vi "Read State com.vi"(8 "error in (no error)":errorcluster, 11 "Master CR in":refnum<class "Master CR.lvclass">) -> (0 "error out":errorcluster, 2 "State com":T1, 3 "Master CR out":refnum<class "Master CR.lvclass">)   [LabVIEW 2021, in "Master CR.lvclass"]
uses:
  Master CR.lvclass
  ctl/Master CR state.ctl
  ctl/CR_Core_State.ctl
  Master CR.lvclass/Master CR.ctl
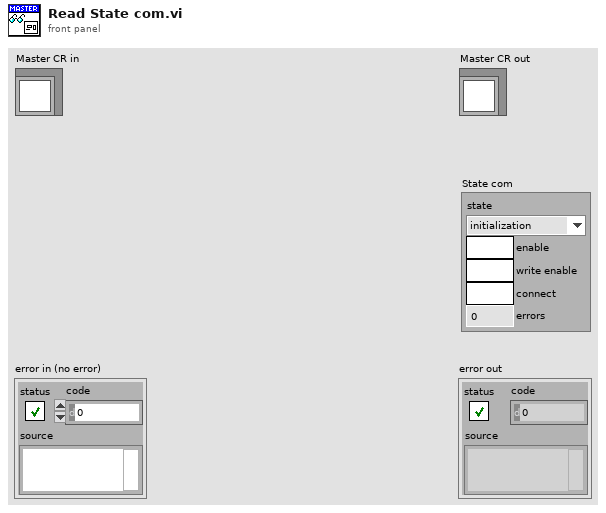
[diagram p1: front panel]
types:
  T1 = typedef "Master CR.lvclass/Master CR state.ctl" = cluster{"state":T2, "enable":bool, "write enable":bool, "connect":bool, "errors":i32}
  T2 = typedef "Master CR.lvclass/CR_Core_State.ctl" = enum8{"initialization", "redefine", "standby", "ping", "connect", "wait to reconnect", "wait to reset timeout", "configure", "requests", "close connection", "stop"}
  T3 = typedef "Master CR.lvclass/MB state.ctl" = cluster{"state":T4, "enable":bool, "write enable":bool, "connect":bool, "errors":i32}
  T4 = typedef "Master CR.lvclass/MB_TCP_State.ctl" = enum8{"initialization", "redefine", "standby", "ping", "connect", "wait to reconnect", "wait to reset timeout", "configure", "requests", "close connection", "stop"}
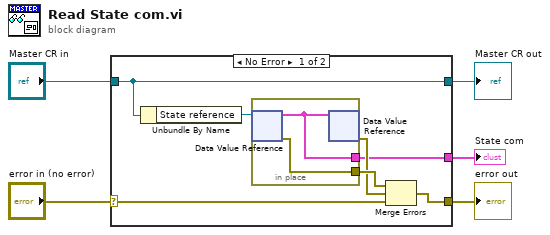
[diagram p0: block diagram]
diagram:
  n1 = case shown="No Error" "error in (no error)" {
    selector: "error in (no error)" -> [w9 w16]
    tunnel: [w6 w16] -> w4
    tunnel: "Master CR in" -> [w8 w15]
    tunnel: [w8 w15] -> w2
    tunnel: [w7 _] -> w1
    frame No Error {
      n2 = Unbundle By Name(w8) -> ("State reference"=w12:refnum<data-value>)
      n3 = in-place {
        in-place-border: [w14] -> w11
        in-place-border: [w13] -> w7
        n4 = in-place-dvr #1(w12) -> (w13:T3, w14:errorcluster)
        n5 = in-place-dvr #1(w13) -> (w10:errorcluster)  [unwired: 1 out]
      }
      n6 = Merge Errors(w11, w10, w9) -> (w6:errorcluster)
    }
    frame Error {
    }
  }
  "error out" <- w4
  "Master CR out" <- w2
  "State com" <- w1
